vi "Imageto64.vi"(11 "path to PNG file":path=path "C:/Users/alan0/Desktop/test.png") -> (3 "Base64 String":string)   [LabVIEW 2021]
uses:
  <vilib>/wsapi/NI_WebServices.lvlib
panel:
  out "Image":T1(plugin-control)
  out "png data":string
  out "FileString":string
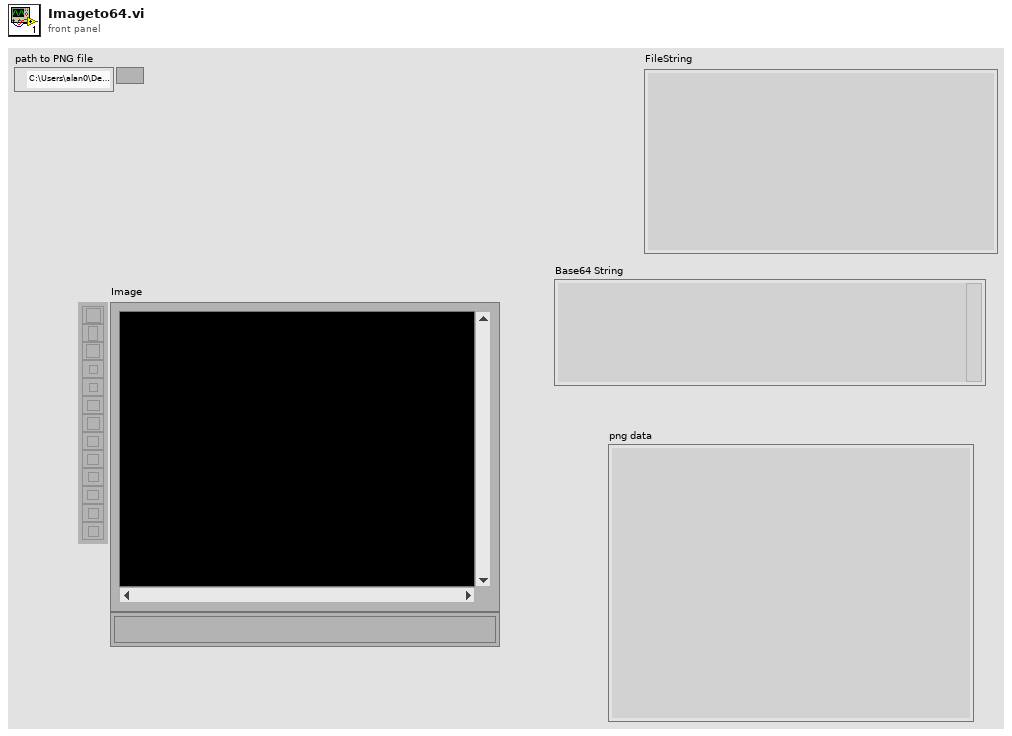
[diagram p1: front panel]
types:
  T1 = typedef "IMAQ Image.ctl" = refnum<image>
  T2 = typedef "imagedata.ctl" = cluster{"image type":i32, "image depth":i32, "image":u8[], "mask":u8[], "colors":u32[], "Rectangle":cluster{"left":i16, "top":i16, "right":i16, "bottom":i16}}
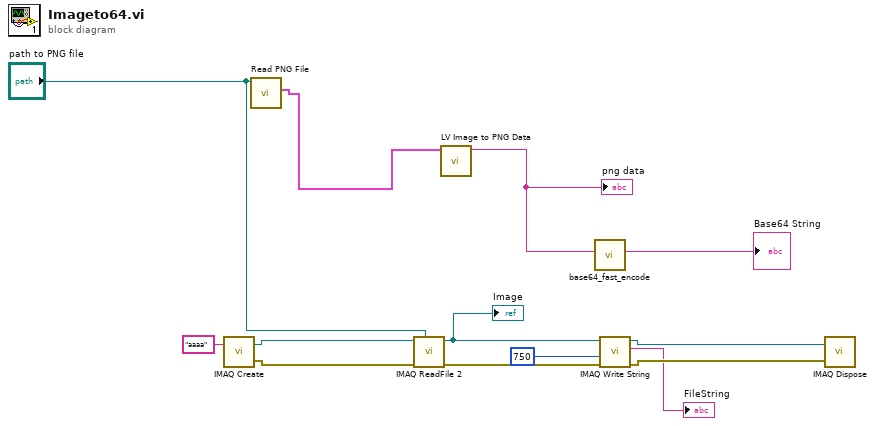
[diagram p0: block diagram]
diagram:
  n1 = call "IMAQ Create"("Image Name"="aaaa") -> ("New Image"=w10:T1, "error out"=w9:errorcluster)  [unwired: 4 in]
  n2 = call <vilib>:"Read PNG File.vi"("path to PNG file"="path to PNG file") -> ("image data"=w11:T2)  [unwired: 8 in, 2 out]
  n3 = call "IMAQ ReadFile 2"("File Path"="path to PNG file", "error in (no error)"=w9, "Image"=w10) -> ("error out"=w1:errorcluster, "Image Out"=w2:T1)  [unwired: 4 in, 3 out]
  "Image" <- w2
  n4 = call <vilib>:"LV Image to PNG Data.vi"("image data"=w11) -> ("png data"=w13:string)  [unwired: 9 in, 1 out]
  "png data" <- w13
  n5 = call "base64_fast_encode.vi"("string in (not encoded)"=w13) -> ("string out (base64-encoded)"=→"Base64 String":string)  [unwired: 9 in, 1 out]
  n6 = call-poly "IMAQ Write String"("error in (no error)"=w1, "Image Quality"=u32 750, "Image"=w2) -> ("error out"=w7:errorcluster, "FileString"=→"FileString":string, "Image Out (duplicate)"=w8:T1)  [unwired: 6 in]
  n7 = call "IMAQ Dispose"("Image"=w8, "error in (no error)"=w7) -> ()  [unwired: 4 in, 1 out]
